vi "ErrorHandler.vi"(0 "Error Message":string, 5 "code":i32, 11 "Error In":errorcluster) -> (15 "Error Out":errorcluster)   [LabVIEW 2013]
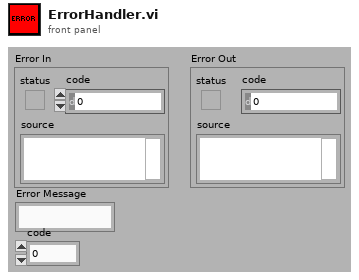
[diagram p1: front panel]
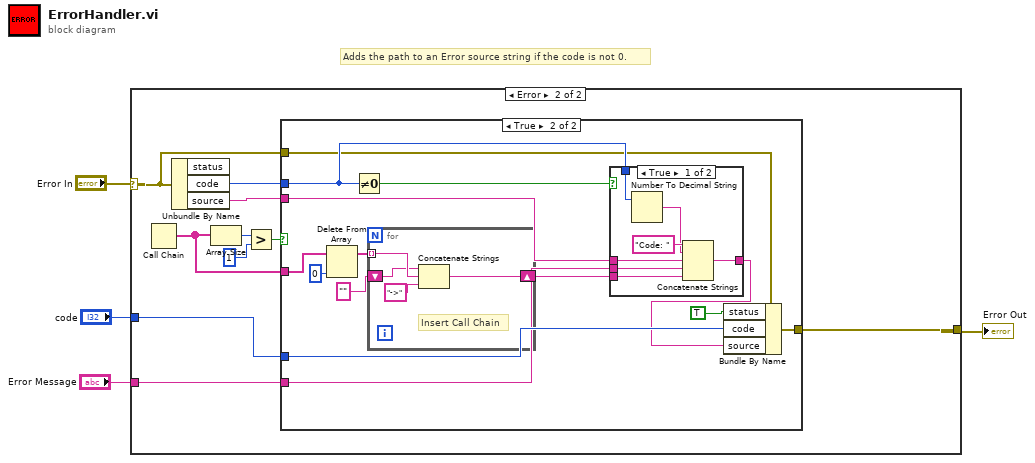
[diagram p0: block diagram]
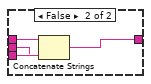
[diagram p4: hidden frame]
diagram:
  # "Adds the path to an Error source string if the code is not 0."
  n1 = case shown="Error" "Error In" {
    selector: "Error In" -> [w5 w6]
    tunnel: "code" -> [_ w9]
    tunnel: "Error Message" -> [_ w8]
    tunnel: [w5 w7] -> w1
    frame No Error {
    }
    frame Error {
      n2 = Call Chain() -> (call chain=w14:string[])
      n3 = Unbundle By Name(w6) -> ("code"=w10:i32, "source"=w11:string)  [unwired: 1 out]
      n4 = Array Size(array=w14) -> (size(s)=w12:i32)
      n5 = Greater?(x=w12, y=1) -> (0:w15:bool)
      n6 = case shown="True" w15 {
        tunnel: w14 -> [_ w30]
        tunnel: w11 -> [_ w26]
        tunnel: w10 -> [_ w24]
        tunnel: w9 -> [_ w23]
        tunnel: w8 -> [_ w19]
        tunnel: [w16 w22] -> w7
        tunnel: w6 -> [w16 w21]
        frame False {
        }
        frame True {
          n7 = Delete From Array(array=w30, index=0) -> (array with subset deleted=w28:string[])  [unwired: 1 in, 1 out]
          n8 = Not Equal To 0?(x=w24) -> (x != 0?=w25:bool)
          n9 = for {
            tunnel: w28 -> [w45] mode=indexing
            shift-right: [w44] -> w20
            shift-left: "" -> [w43]
            # "Insert Call Chain"
            n10 = Concatenate Strings(w43, w45, "->") -> (w44:string)
          }
          n11 = case shown="True" w25 {
            tunnel: w26 -> [w37 w41]
            tunnel: w24 -> [w35 _]
            tunnel: w20 -> [w31 w39]
            tunnel: w19 -> [w33 w38]
            tunnel: [w32 w40] -> w18
            frame True {
              n12 = Number To Decimal String(number=w35) -> (decimal integer string=w34:string)  [unwired: 1 in]
              n13 = Concatenate Strings("Code: " ("string"), w34, w37, w33, w31) -> (w32:string)
            }
            frame False {
              n14 = Concatenate Strings(w41, w39, w38) -> (w40:string)
            }
          }
          n15 = Bundle By Name(cluster=w21, "status"=TRUE, "code"=w23, "source"=w18) -> (w22:errorcluster)
        }
      }
    }
  }
  "Error Out" <- w1
